vi "proba_neo_kinect.vi"() -> ()   [LabVIEW 2012]
panel:
  out "s? t:f":dbl
  in  "x":dbl(slide) scale=-2.0..2.0
  in  "y":dbl(slide) scale=-2.0..4.0
  in  "gear":i32(knob)=12 scale=20.0..1.0
  out "Jobb":dbl(slide) scale=-2.0..2.0
  out "Bal":dbl(slide) scale=-2.0..2.0 scale format="%0#1_1g"
  out "XY Graph":cluster{dbl, dbl}[](graph)
  in  "stop":bool
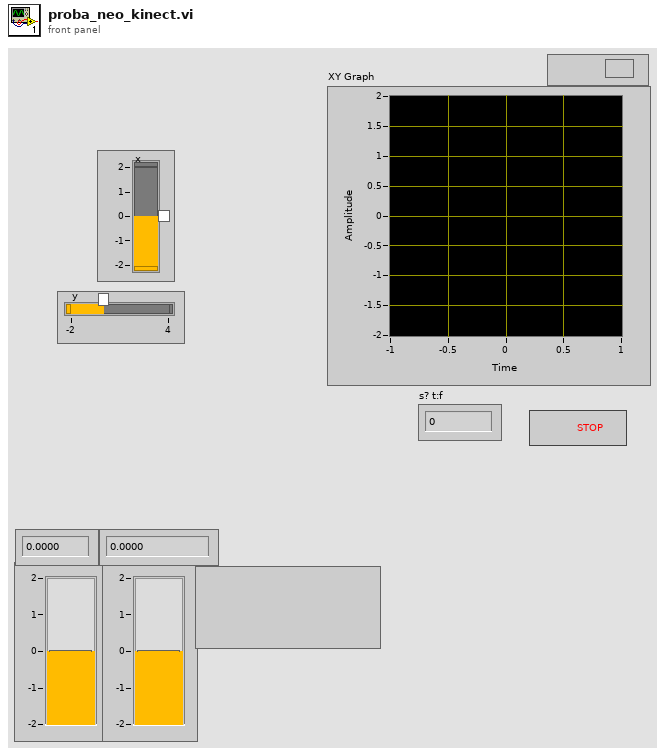
[diagram p1: front panel]
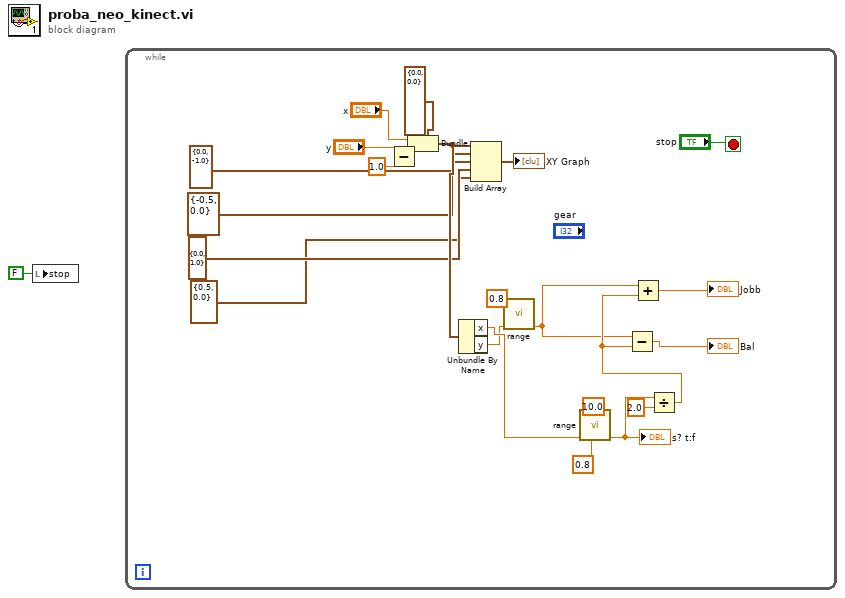
[diagram p0: block diagram]
diagram:
  n1 = local write "stop"(FALSE ("stop")) -> ()
  n2 = while {
    stop <- "stop" stop-if-true
    n3 = Subtract(x="y", y=1.0) -> (x-y=w18:dbl)
    n4 = Bundle(cluster=cluster{"x":dbl, "y":dbl} {"x"=0.0, "y"=0.0}, "x"="x", "y"=w18) -> (w23:cluster{"x":dbl, "y":dbl})
    n5 = Unbundle By Name(w23) -> ("x"=w3:dbl, "y"=w2:dbl)
    n6 = Build Array(w23, cluster{"Numeric":dbl, "Numeric":dbl} {"Numeric"=0.0, "Numeric"=-1.0} ("element"), cluster{"Numeric":dbl, "Numeric":dbl} {"Numeric"=-0.5, "Numeric"=0.0} ("element"), cluster{"Numeric":dbl, "Numeric":dbl} {"Numeric"=0.0, "Numeric"=1.0} ("element"), cluster{"Numeric":dbl, "Numeric":dbl} {"Numeric"=0.5, "Numeric"=0.0} ("element")) -> (→"XY Graph":cluster{"Numeric":dbl, "Numeric":dbl}[])
    n7 = call "range.vi"("also"=0.8, "n"=w2) -> ("n2"=w5:dbl)  [unwired: 9 in]
    n8 = call "range.vi"("felso"=10.0 ("lower limit"), "also"=0.8 ("upper limit"), "n"=w3) -> ("n2"=w8:dbl)  [unwired: 8 in]
    "s? t:f" <- w8
    n9 = Divide(x=w8, y=2.0) -> (x/y=w6:dbl)
    n10 = Subtract(x=w5, y=w6) -> (x-y=→"Bal":dbl)
    n11 = Add(x=w5, y=w6) -> (x+y=→"Jobb":dbl)
  }
